vi "Run Panel.vi"(6 "Dock Event":refnum<user-event>, 7 "Pane Offset":cluster{"Height":u32, "Numeric":u32}, 8 "error in (no error)":errorcluster, 9 "Variant Repository Out":variant, 10 "Move Event":refnum<user-event>, 11 "Pane in":refnum<vi>) -> (0 "error out":errorcluster, 3 "Panel VI Ref":refnum<vi>)   [LabVIEW 2011]
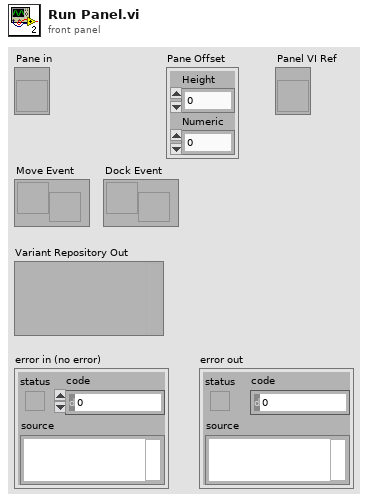
[diagram p1: front panel]
types:
  T1 = typedef "Semaphore RefNum" = refnum<k1>
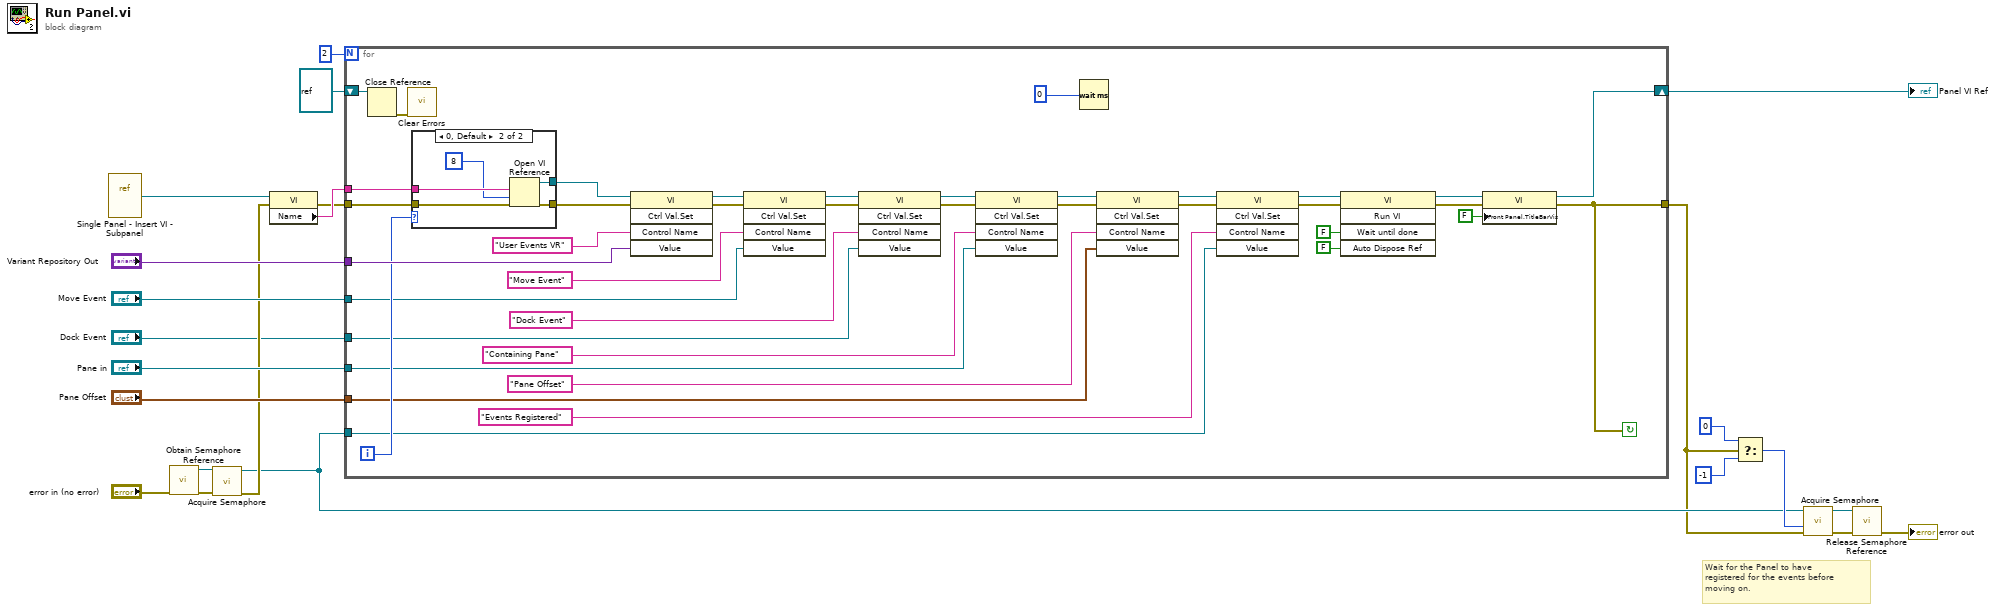
[diagram p0: block diagram]
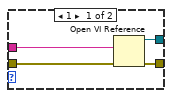
[diagram p2: hidden frame]
diagram:
  # "Wait for the Panel to have registered for the events before moving on."
  n1 = vi-ref "Single Panel - Insert VI - Subpanel.vi"() -> (w17:refnum<vi>)
  n2 = call <vilib>:"Obtain Semaphore Reference.vi"("error in (no error)"="error in (no error)") -> ("error out"=w10:errorcluster, "semaphore"=w11:T1)  [unwired: 4 in, 1 out]
  n3 = call <vilib>:"Acquire Semaphore.vi"("error in (no error)"=w10, "semaphore"=w11) -> ("error out"=w8:errorcluster, "semaphore out"=w4:T1)  [unwired: 3 in, 1 out]
  n4 = property class="VI"(reference=w17, error in=w8) -> (error out=w15:errorcluster, "Name"=w16:string)  [unwired: 1 out]
  n5 = for {
    N: 2 -> [_]
    tunnel: "Variant Repository Out" -> [w60]
    tunnel: w15 -> [w56]
    tunnel: [w42] -> w3
    shift-right: [w43] -> w21
    shift-left: refnum<vi> refnum ("vi reference") -> [w52]
    tunnel: w16 -> [w50]
    tunnel: w4 -> [w47]
    tunnel: "Pane in" -> [w40]
    tunnel: "Pane Offset" -> [w34]
    tunnel: "Move Event" -> [w30]
    tunnel: "Dock Event" -> [w24]
    i -> [w53]
    stop <- w42 continue-if-true
    n6 = Close Reference(reference=w52) -> (error out=w51:errorcluster)  [unwired: 1 in]
    n7 = call <vilib>:"Clear Errors.vi"("error in (no error)"=w51) -> ()  [unwired: 6 in, 1 out]
    n8 = case shown="0, Default" w53 {
      tunnel: [w65 w71] -> w62
      tunnel: [w66 w70] -> w61
      tunnel: w50 -> [w63 w69]
      tunnel: w56 -> [w64 w68]
      frame 1 {
        n9 = Open VI Reference(vi path=w63, error in (no error)=w64) -> (vi reference=w66:refnum<vi>, error out=w65:errorcluster)  [unwired: 4 in]
      }
      frame 0, Default {
        n10 = Open VI Reference(vi path=w69, options=8, error in (no error)=w68) -> (vi reference=w70:refnum<vi>, error out=w71:errorcluster)  [unwired: 3 in]
      }
    }
    n11 = invoke class="VI" method="Ctrl Val.Set"(reference=w61, error in=w62, "Control Name"="User Events VR", "Value"=w60) -> (reference out=w31:refnum<vi>, error out=w41:errorcluster)  [unwired: 1 in, 3 out]
    n12 = invoke class="VI" method="Ctrl Val.Set"(reference=w31, error in=w41, "Control Name"="Move Event", "Value"=w30) -> (reference out=w27:refnum<vi>, error out=w32:errorcluster)  [unwired: 1 in, 3 out]
    n13 = invoke class="VI" method="Ctrl Val.Set"(reference=w27, error in=w32, "Control Name"="Dock Event", "Value"=w24) -> (reference out=w26:refnum<vi>, error out=w28:errorcluster)  [unwired: 1 in, 3 out]
    n14 = invoke class="VI" method="Ctrl Val.Set"(reference=w26, error in=w28, "Control Name"="Containing Pane", "Value"=w40) -> (reference out=w38:refnum<vi>, error out=w37:errorcluster)  [unwired: 1 in, 3 out]
    n15 = Wait (ms)(milliseconds to wait=u32 0) -> ()  [unwired: 1 out]
    n16 = invoke class="VI" method="Ctrl Val.Set"(reference=w38, error in=w37, "Control Name"="Pane Offset", "Value"=w34) -> (reference out=w36:refnum<vi>, error out=w35:errorcluster)  [unwired: 1 in, 3 out]
    n17 = invoke class="VI" method="Ctrl Val.Set"(reference=w36, error in=w35, "Control Name"="Events Registered", "Value"=w47) -> (reference out=w44:refnum<vi>, error out=w48:errorcluster)  [unwired: 1 in, 3 out]
    n18 = invoke class="VI" method="Run VI"(reference=w44, error in=w48, "Wait until done"=FALSE ("Wait Until Done"), "Auto Dispose Ref"=FALSE ("Auto Dispose Reference")) -> (reference out=w55:refnum<vi>, error out=w54:errorcluster)  [unwired: 1 in, 3 out]
    n19 = property class="VI"(reference=w55, error in=w54, "Front Panel.TitleBarVis"=FALSE ("Front Panel Window:Title Bar Visible")) -> (reference out=w43:refnum<vi>, error out=w42:errorcluster)
  }
  "Panel VI Ref" <- w21
  n20 = Select(t=0, s=w3, f=-1 ("ms timeout (-1)")) -> (s? t:f=w5:i32)
  n21 = call <vilib>:"Acquire Semaphore.vi"("error in (no error)"=w3, "ms timeout (-1)"=w5, "semaphore"=w4) -> ("error out"=w7:errorcluster, "semaphore out"=w6:T1)  [unwired: 2 in, 1 out]
  n22 = call <vilib>:"Release Semaphore Reference.vi"("error in (no error)"=w7, "semaphore"=w6) -> ("error out"=→"error out":errorcluster)  [unwired: 8 in, 1 out]
